vi "Data Access.vi"(8 "error in (no error)":errorcluster, 10 "Data Access Handler":refnum<class "Data Access Handler.lvclass">, 11 "DMM Triggered Measure Msg in":refnum<class "DMM Triggered Measure Msg.lvclass">) -> (0 "error out":errorcluster, 3 "DMM Triggered Measure Msg out":refnum<class "DMM Triggered Measure Msg.lvclass">)   [LabVIEW 2020, in "DMM Msg.lvlib" / "DMM Triggered Measure Msg.lvclass"]
doc: "Expose class private data to the front panel while letting the Data Access Handler class act on the data."
uses:
  DMM Triggered Measure Msg.lvclass
  C:/Current projects/WS/PPL/HDH.Actor Framework.Core.Msg.lvlibp/Flex Msg/Flex Msg.lvclass
  PPL/HDH.Actor Framework.Core.Msg.lvlibp/Flex Msg/Data Access Handlers/Data Access Handler/Data Access Handler.lvclass
  PPL/HDH.Actor Framework.Core.Publisher.lvlibp/Messages/Response Msg/Response Core/Controls/Ctl_SendFunction.ctl
  DMM Triggered Measure Msg.lvclass/DMM Triggered Measure Msg.ctl
  PPL/HDH.Actor Framework.Core.Instrument Handler.lvlibp/Messages/Instrument Msg/Instrument Msg.lvclass
  C:/Current projects/WS/PPL/HDH.Actor Framework.Core.Instrument Handler.lvlibp/Messages/Instrument Msg/Instrument Msg.lvclass
  PPL/HDH.Actor Framework.Core.Publisher.lvlibp
panel:
  in  "Publish?":bool=TRUE
  in  "Check Range?":bool=TRUE
  in  "Restore Range if Changed?":bool=TRUE
  in  "Max Time(ms)":i32=-1
  in  "Measurements to Acquire":i32=1
  in  "Message Priority":enum16{"Low", "Normal", "High"}(ring)=enum."Normal"
  in  "Timeout if Waiting":i32=-1
  in  "Send Function":T1=enum."Await Reply"
  in  "Cancel":bool
  in  "OK":bool
  # "Send details"
  # "Measure details"
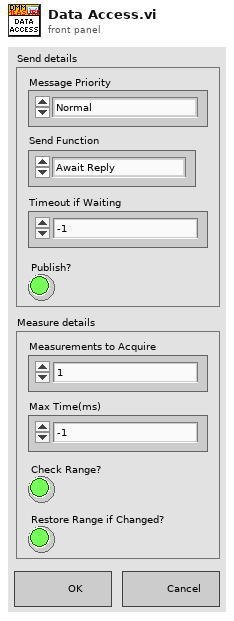
[diagram p1: front panel]
types:
  T1 = typedef "HDH.Actor Framework.Core.Publisher.lvlibp/Ctl_SendFunction.ctl" = enum16{"Send and Forget", "Request Reply", "Await Reply"}
  T2 = typedef "HDH.Actor Framework.Core.Actor.lvlibp/Message Enqueuer.lvclass/Message Priority.ctl" = enum16{"Low", "Normal", "High"}
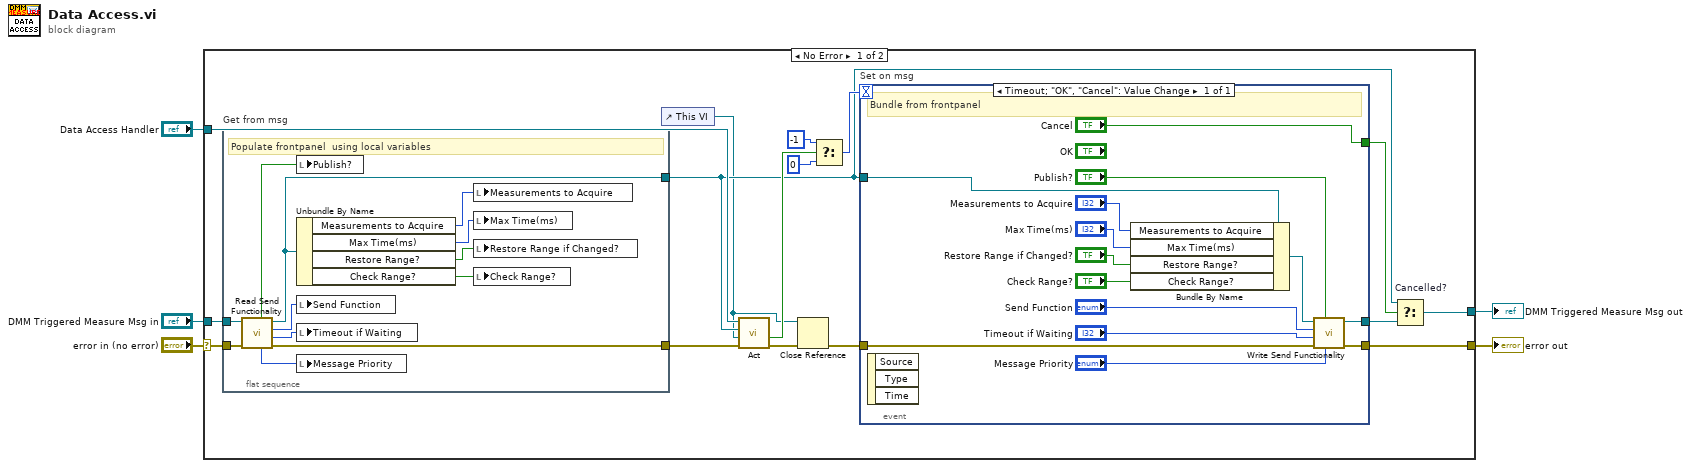
[diagram p0: block diagram]
diagram:
  n1 = case shown="No Error" "error in (no error)" {
    selector: "error in (no error)" -> [w21 w49]
    tunnel: [w14 w49] -> w4
    tunnel: [w9 w48] -> w2
    tunnel: "DMM Triggered Measure Msg in" -> [w12 w48]
    tunnel: "Data Access Handler" -> [w20 _]
    frame No Error {
      n2 = flat-sequence "Get from msg" {
        tunnel: w21 -> [w46]
        tunnel: [w44] -> w7
        tunnel: w12 -> [w47]
        tunnel: [w45] -> w19
        frame #0 {
          # "Populate frontpanel  using local variables"
          n3 = call "Read Send Functionality.vi"("error in (no error)"=w46, "Instrument Msg in"=w47) -> ("error out"=w45:errorcluster, "Timeout if Waiting"=w42:i32, "Send Function"=w43:T1, "Instrument Msg out"=w44:refnum<class "DMM Triggered Measure Msg.lvclass">, "Message Priority"=w41:T2, "Publish Data?"=w36:bool)  [unwired: 4 in]
          n4 = local write "Publish?"(w36) -> ()
          n5 = Unbundle By Name(w44) -> ("Measurements to Acquire"=w40:i32, "Max Time(ms)"=w39:i32, "Restore Range?"=w38:bool, "Check Range?"=w37:bool)
          n6 = local write "Send Function"(w43) -> ()
          n7 = local write "Timeout if Waiting"(w42) -> ()
          n8 = local write "Message Priority"(w41) -> ()
          n9 = local write "Measurements to Acquire"(w40) -> ()
          n10 = local write "Max Time(ms)"(w39) -> ()
          n11 = local write "Restore Range if Changed?"(w38) -> ()
          n12 = local write "Check Range?"(w37) -> ()
        }
      }
      n13 = control-ref of="This VI"() -> (w6:refnum<vi>)
      n14 = call-dynamic "Act.vi"("error in (no error)"=w19, "VI Refnum in"=w6, "Flex Msg type"=w7, "Data Access Handler in"=w20) -> ("error out"=w11:errorcluster, "Await user action?"=w18:bool)  [unwired: 5 in, 1 out]
      n15 = Close Reference(reference=w6, error in (no error)=w11) -> (error out=w13:errorcluster)
      n16 = Select(t=-1, s=w18, f=0 ("t")) -> (s? t:f=w15:i32)
      n17 = event "Set on msg" shown="[0] Timeout;  \"OK\", \"Cancel\": Value Change" {
        selector: _ -> [_]
        dyn-events: _ -> [_]
        timeout: w15 -> [_]
        tunnel: [w30] -> w14
        tunnel: w13 -> [w31]
        tunnel: ["Cancel"] -> w10
        tunnel: [w33] -> w8
        tunnel: w7 -> [w34]
        event Timeout; "OK", "Cancel": Value Change {
          # "Bundle from frontpanel"
          n18 = event-data() -> ()  [unwired: 1 in, 3 out]
          n19 = Bundle By Name(cluster=w34, "Measurements to Acquire"="Measurements to Acquire", "Max Time(ms)"="Max Time(ms)", "Restore Range?"="Restore Range if Changed?", "Check Range?"="Check Range?") -> (w32:refnum<class "DMM Triggered Measure Msg.lvclass">)
          n20 = call "Write Send Functionality.vi"("Message Priority(Normal)"="Message Priority", "Publish Data?(T)"="Publish?", "error in (no error)"=w31, "Timeout if Waiting(-1ms)"="Timeout if Waiting", "Send Function(Await Reply)"="Send Function", "Instrument Msg in"=w32) -> ("error out"=w30:errorcluster, "Instrument Msg out"=w33:refnum<class "DMM Triggered Measure Msg.lvclass">)  [unwired: 4 in]
        }
      }
      n21 = Select "Cancelled?"(t=w7, s=w10, f=w8) -> (s? t:f=w9:refnum<class "DMM Triggered Measure Msg.lvclass">)
    }
    frame Error {
    }
  }
  "error out" <- w4
  "DMM Triggered Measure Msg out" <- w2
